vi "Create.vi"(7 "Direction":T1, 8 "error in (no error)":errorcluster, 9 "Custom Config Data":u8[](array[numeric]), 10 "Name":string, 11 "CIFTag in":refnum<class "CIFTagU64.lvclass">) -> (0 "error out":errorcluster, 3 "CIFTag out":refnum<class "CIFTagU64.lvclass">)   [LabVIEW 2021, in "CIFTagU64.lvclass"]
uses:
  CIFTagU64.lvclass
  D:/dev/CIF-LVCore/src/Channels/CIFChannels/CIFChannels.lvclass
  D:/dev/CIF-LVCore/src/Channels/CIFTag/CIFTag/CIFTag.lvclass
  CIFChannels/Typedef/Direction.ctl
  CIFChannels/Typedef/Disconnect Behavior.ctl
  CIFChannels/CIFChannels.lvclass/CIFChannels.ctl
  CIFChannels/Typedef/Channel State.ctl
  CIFTagU64.lvclass/CIFTagU64.ctl
  CIFTag/CIFTag.lvclass/CIFTag.ctl
  05ae5bac-bc51-4698-a6dd-26343cf35d94.vi
  484728b7-4164-4b2b-b47a-7b7a48845692.vi
  a7aee11b-fbf7-4338-a5a4-084a4d8dd976.vi
  78e3d3e5-03e0-4404-95f9-7bd2f40b88e3.vi
  CIFChannels/Accessors/Write Channel State.vi
  CIFTag/Accessors/Write CIF Channel.vi
  CIFChannels/SubVIs/Get Type from Class.vi
  CIFChannels/Accessors/Write Type.vi
  CIFChannels/Accessors/Write Channel Class.vi
  CIFChannels/Accessors/Write Direction.vi
  CIFChannels/Accessors/Write Disconnect Behavior.vi
  CIFChannels/Accessors/Write Name.vi
  CIFChannels/Accessors/Write Custom Config Data.vi
  <vilib>/CIFChannels/SubVIs/Add Error.vi
  05ae5bac-bc51-4698-a6dd-26343cf35d94.vi/c28b0ead-42ad-4072-80a2-aca7f2bd7ce3.vi
  <vilib>/CIFChannels/SubVIs/CIFServices Fill In Error Info Ex.vi
  <vilib>/CIFChannels/SubVIs/Get dll Path.vi
  484728b7-4164-4b2b-b47a-7b7a48845692.vi/4bc1c15b-36ab-481f-b8dd-c64075ce723a.vi
  484728b7-4164-4b2b-b47a-7b7a48845692.vi/d83cb72b-7713-41fc-a3d1-682de79cf574.vi
  a7aee11b-fbf7-4338-a5a4-084a4d8dd976.vi/c28b0ead-42ad-4072-80a2-aca7f2bd7ce3.vi
  78e3d3e5-03e0-4404-95f9-7bd2f40b88e3.vi/4bc1c15b-36ab-481f-b8dd-c64075ce723a.vi
  <vilib>/CIFChannels/SubVIs/Append Error Location.vi
  CIFChannels/CIFChannels.lvclass
  D:/dev/CIF-LVCore/src/Channels/CIFTag/U64/CIFTagU64.lvclass
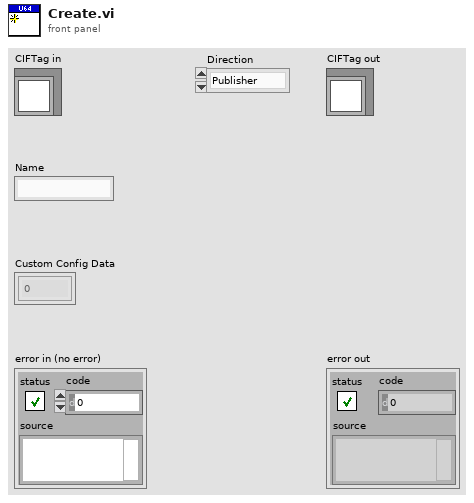
[diagram p1: front panel]
types:
  T1 = typedef "CIFChannels.lvclass/Direction.ctl" = enum16{"Publisher", "Subscriber"}
  T2 = typedef "CIFChannels.lvclass/Disconnect Behavior.ctl" = enum16{"Default value", "Last value", "Error with default"}
  T3 = typedef "CIFChannels.lvclass/Channel State.ctl" = enum16{"Creating", "Disconnected", "Connecting", "Connected", "Destroyed"}
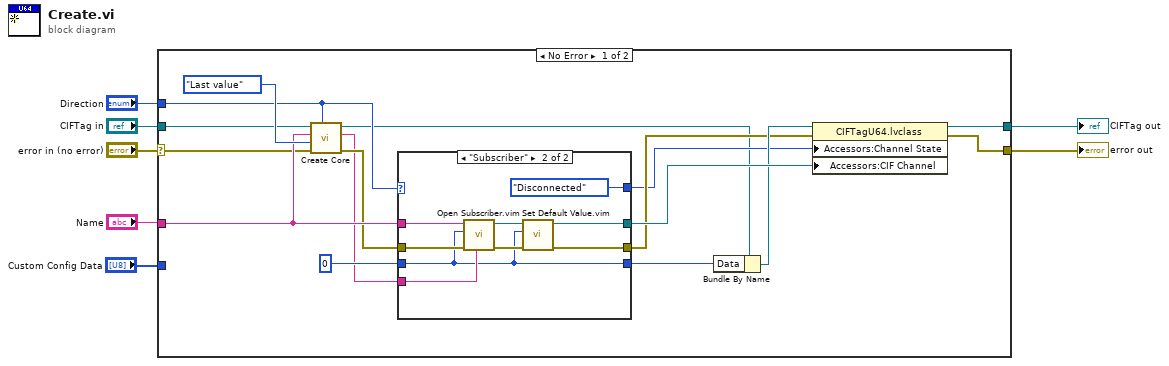
[diagram p0: block diagram]
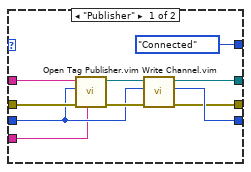
[diagram p2: hidden frame]
diagram:
  n1 = case shown="No Error" "error in (no error)" {
    selector: "error in (no error)" -> [w8 w44]
    tunnel: [w22 w44] -> w2
    tunnel: [w15 w43] -> w3
    tunnel: "CIFTag in" -> [w14 w43]
    tunnel: "Name" -> [w21 _]
    tunnel: "Direction" -> [w13 _]
    tunnel: "Custom Config Data" -> [_ _]
    frame No Error {
      n2 = call "Create Core.vi"("Direction"=w13, "error in (no error)"=w8, "Disconnect Behavior"=Disconnect_Behavior."Last value", "Name"=w21, "CIFChannels in"=w14) -> ("error out"=w20:errorcluster, "Channel Type"=w9:string, "CIFChannels out"=w11:refnum<class "CIFTagU64.lvclass">)  [unwired: 4 in]
      n3 = case shown="\"Subscriber\"" w13 {
        tunnel: w21 -> [w33 w41]
        tunnel: w20 -> [w32 w40]
        tunnel: [w29 w37] -> w19
        tunnel: u64 0 ("Default Value") -> [w28 w34]
        tunnel: [w27 w34] -> w17
        tunnel: [w26 w36] -> w16
        tunnel: w9 -> [w25 w35]
        tunnel: [Channel_State."Connected" ("Channel State") Channel_State."Disconnected" ("Channel State")] -> w12
        frame "Publisher" {
          n4 = call "Open Tag Publisher.vim"("Channel Type Description"=w25, "error in"=w32, "Input Type"=w28, "Channel Name"=w33) -> ("error out"=w30:errorcluster, "CIF Channel"=w31:refnum<k21>)  [unwired: 6 in]
          n5 = call "Write Channel.vim"("error in"=w30, "Data in"=w28, "CIF Channel in"=w31) -> ("error out"=w26:errorcluster, "Data out"=w27:u64, "CIF Channel out"=w29:refnum<k21>)  [unwired: 5 in, 1 out]
        }
        frame "Subscriber" {
          n6 = call "Open Subscriber.vim"("Channel Type Description"=w35, "error in"=w40, "Input Type"=w34, "Channel Name"=w41) -> ("error out"=w39:errorcluster, "CIF Channel"=w38:refnum<k21>)  [unwired: 6 in]
          n7 = call "Set Default Value.vim"("error in"=w39, "Data in"=w34, "CIF Channel in"=w38) -> ("error out"=w36:errorcluster, "CIF Channel out"=w37:refnum<k21>)  [unwired: 7 in]
        }
      }
      n8 = Bundle By Name(cluster=w11, "Data"=w17) -> (w18:refnum<class "CIFTagU64.lvclass">)
      n9 = property class="CIFTagU64.lvclass"(reference=w18, error in=w16, "Accessors:Channel State"=w12, "Accessors:CIF Channel"=w19) -> (reference out=w15:refnum<class "CIFTagU64.lvclass">, error out=w22:errorcluster)
    }
    frame Error {
    }
  }
  "error out" <- w2
  "CIFTag out" <- w3
